vi "Python_Status.vi"(8 "error in (no error)":errorcluster) -> (0 "error out":errorcluster, 1 "return value":i32)   [LabVIEW 2021]
doc: "This example demonstrates how to call a Python function and pass integers as arguments. It uses a python function to compute the sum of two integers."
uses:
  Global_Variables.vi
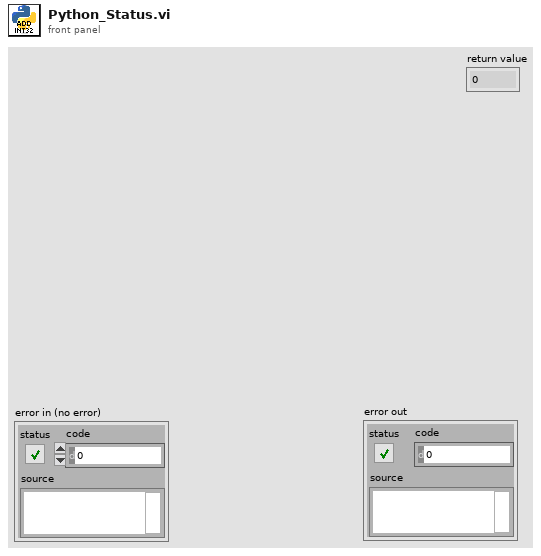
[diagram p1: front panel]
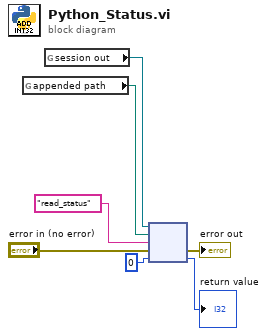
[diagram p0: block diagram]
diagram:
  n1 = global read "Global_Variables.vi" "appended path"() -> (w2:path)
  n2 = global read "Global_Variables.vi" "session out"() -> (w1:refnum<k35>)
  n3 = node(w1, w2, "read_status" ("function name"), "error in (no error)", 0) -> (→"error out":errorcluster, →"return value":i32)  [unwired: 3 out]
